vi "Remove Duplicates.vi"(1 "Array In":errorcluster[](array[cluster])) -> (0 "Array Out":errorcluster[](array[cluster]))   [LabVIEW 2020, in "Instrument Addon Protections Unit Tests.lvclass"]
uses:
  Instrument Addon Protections Unit Tests.lvclass
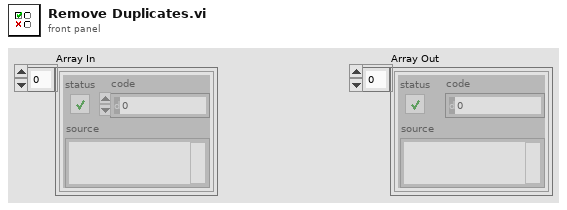
[diagram p1: front panel]
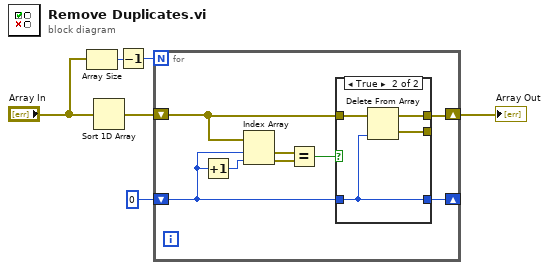
[diagram p0: block diagram]
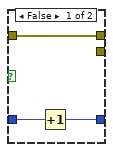
[diagram p2: hidden frame]
diagram:
  n1 = Array Size(array="Array In") -> (size(s)=w2:i32)
  n2 = Sort 1D Array(array="Array In") -> (sorted array=w5:errorcluster[])
  n3 = Decrement(x=w2) -> (x-1=w1:i32)
  n4 = for {
    N: w1 -> [_]
    shift-right: [w13] -> w6
    shift-left: w5 -> [w14]
    shift-right: [w8] -> _
    shift-left: 0 -> [w7]
    n5 = Increment(x=w7) -> (x+1=w9:i32)
    n6 = Index Array(array=w14, index #1=w7, index #2=w9) -> (element #1=w12:errorcluster, element #2=w11:errorcluster)
    n7 = Equal?(x=w12, y=w11) -> (x = y?=w10:bool)
    n8 = case shown="True" w10 {
      tunnel: w14 -> [w17 w21]
      tunnel: [w17 w20] -> w13
      tunnel: w7 -> [w16 w19]
      tunnel: [w15 w19] -> w8
      tunnel: [_ w18] -> _
      frame False {
        n9 = Increment(x=w16) -> (x+1=w15:i32)
      }
      frame True {
        n10 = Delete From Array(array=w21, index=w19) -> (deleted portion=w18:errorcluster, array with subset deleted=w20:errorcluster[])  [unwired: 1 in]
      }
    }
  }
  "Array Out" <- w6
